vi "HandleObservation.vi"(8 "error in (no error)":errorcluster, 11 "S4ACS_GUI in":refnum<class "S4ACS_GUI.lvclass">) -> (0 "error out":errorcluster, 3 "S4ACS_GUI out":refnum<class "S4ACS_GUI.lvclass">)   [LabVIEW 2018, in "S4ACS_GUI.lvclass"]
uses:
  S4ACS_GUI.lvclass
  S4ACS_GUI.lvclass/S4ACS_GUI.ctl
  Server/Server.lvclass/Server.ctl
  Acquisition/Acquisition.lvclass
  C:/Users/observer/Desktop/Sparc4GUI/SPARC4_GUI/Server/Server.lvclass
  Server/Server.lvclass
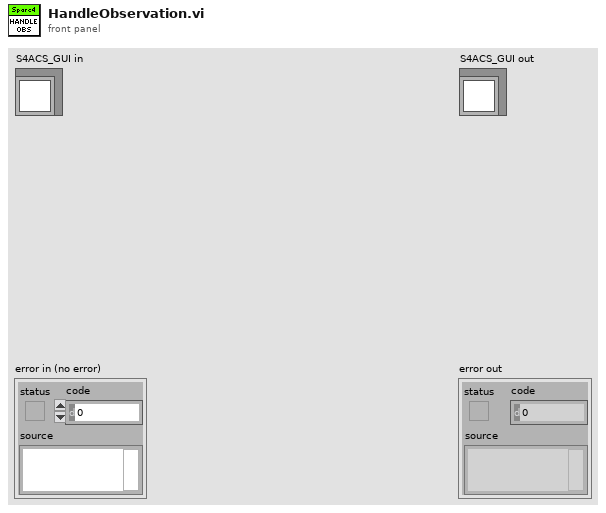
[diagram p1: front panel]
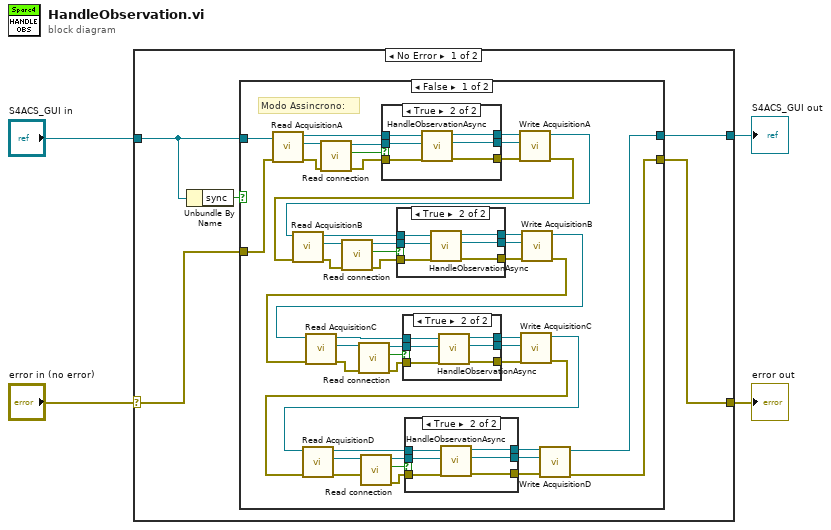
[diagram p0: block diagram]
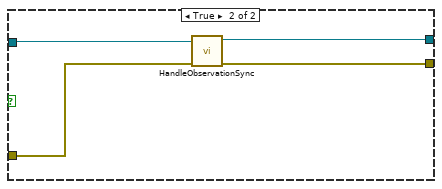
[diagram p6: hidden frame]
diagram:
  n1 = case shown="No Error" "error in (no error)" {
    selector: "error in (no error)" -> [w6 w97]
    tunnel: [w5 w97] -> w3
    tunnel: [w8 w96] -> w1
    tunnel: "S4ACS_GUI in" -> [w9 w96]
    frame No Error {
      n2 = Unbundle By Name(w9) -> ("sync"=w7:bool)
      n3 = case shown="False" w7 {
        tunnel: w9 -> [w55 w95]
        tunnel: [w47 w94] -> w8
        tunnel: w6 -> [w53 w93]
        tunnel: [w46 w92] -> w5
        frame False {
          # "Modo Assincrono:"
          n4 = call-dynamic "Read AcquisitionA.vi"("error in (no error)"=w53, "S4ACS_GUI in"=w55) -> ("error out"=w38:errorcluster, "Acquisition.lvclass"=w41:refnum<class "Acquisition.lvclass">, "S4ACS_GUI out"=w54:refnum<class "S4ACS_GUI.lvclass">)  [unwired: 7 in]
          n5 = call "Read connection.vi"("error in (no error)"=w38, "Server in"=w41) -> ("error out"=w37:errorcluster, "connection"=w39:bool, "Server out"=w40:refnum<class "Acquisition.lvclass">)  [unwired: 7 in]
          n6 = case shown="True" w39 {
            tunnel: w54 -> [w84 w91]
            tunnel: w40 -> [w85 w90]
            tunnel: w37 -> [w83 w89]
            tunnel: [w84 w88] -> w52
            tunnel: [w85 w87] -> w51
            tunnel: [w83 w86] -> w50
            frame False {
            }
            frame True {
              n7 = call-dynamic "HandleObservationAsync.vi"("error in (no error)"=w89, "Acquisition.lvclass In"=w90, "S4ACS_GUI in"=w91) -> ("error out"=w86:errorcluster, "Acquisition.lvclass Out"=w87:refnum<class "Acquisition.lvclass">, "S4ACS_GUI out"=w88:refnum<class "S4ACS_GUI.lvclass">)  [unwired: 6 in]
            }
          }
          n8 = call-dynamic "Write AcquisitionA.vi"("error in (no error)"=w50, "Acquisition.lvclass"=w51, "S4ACS_GUI in"=w52) -> ("error out"=w49:errorcluster, "S4ACS_GUI out"=w48:refnum<class "S4ACS_GUI.lvclass">)  [unwired: 7 in]
          n9 = call "Read AcquisitionB.vi"("error in (no error)"=w49, "S4ACS_GUI in"=w48) -> ("error out"=w32:errorcluster, "Acquisition.lvclass"=w35:refnum<class "Acquisition.lvclass">, "S4ACS_GUI out"=w36:refnum<class "S4ACS_GUI.lvclass">)  [unwired: 7 in]
          n10 = call "Read connection.vi"("error in (no error)"=w32, "Server in"=w35) -> ("error out"=w31:errorcluster, "connection"=w33:bool, "Server out"=w34:refnum<class "Acquisition.lvclass">)  [unwired: 7 in]
          n11 = case shown="True" w33 {
            tunnel: w36 -> [w75 w82]
            tunnel: w34 -> [w76 w81]
            tunnel: w31 -> [w74 w80]
            tunnel: [w75 w79] -> w28
            tunnel: [w76 w78] -> w29
            tunnel: [w74 w77] -> w30
            frame False {
            }
            frame True {
              n12 = call-dynamic "HandleObservationAsync.vi"("error in (no error)"=w80, "Acquisition.lvclass In"=w81, "S4ACS_GUI in"=w82) -> ("error out"=w77:errorcluster, "Acquisition.lvclass Out"=w78:refnum<class "Acquisition.lvclass">, "S4ACS_GUI out"=w79:refnum<class "S4ACS_GUI.lvclass">)  [unwired: 6 in]
            }
          }
          n13 = call "Write AcquisitionB.vi"("error in (no error)"=w30, "Acquisition.lvclass"=w29, "S4ACS_GUI in"=w28) -> ("error out"=w45:errorcluster, "S4ACS_GUI out"=w44:refnum<class "S4ACS_GUI.lvclass">)  [unwired: 7 in]
          n14 = call-dynamic "Read AcquisitionC.vi"("error in (no error)"=w45, "S4ACS_GUI in"=w44) -> ("error out"=w19:errorcluster, "Acquisition.lvclass"=w20:refnum<class "Acquisition.lvclass">, "S4ACS_GUI out"=w24:refnum<class "S4ACS_GUI.lvclass">)  [unwired: 7 in]
          n15 = call "Read connection.vi"("error in (no error)"=w19, "Server in"=w20) -> ("error out"=w25:errorcluster, "connection"=w26:bool, "Server out"=w27:refnum<class "Acquisition.lvclass">)  [unwired: 7 in]
          n16 = case shown="True" w26 {
            tunnel: w24 -> [w66 w73]
            tunnel: w27 -> [w67 w72]
            tunnel: w25 -> [w65 w71]
            tunnel: [w66 w70] -> w23
            tunnel: [w67 w69] -> w22
            tunnel: [w65 w68] -> w21
            frame False {
            }
            frame True {
              n17 = call-dynamic "HandleObservationAsync.vi"("error in (no error)"=w71, "Acquisition.lvclass In"=w72, "S4ACS_GUI in"=w73) -> ("error out"=w68:errorcluster, "Acquisition.lvclass Out"=w69:refnum<class "Acquisition.lvclass">, "S4ACS_GUI out"=w70:refnum<class "S4ACS_GUI.lvclass">)  [unwired: 6 in]
            }
          }
          n18 = call-dynamic "Write AcquisitionC.vi"("error in (no error)"=w21, "Acquisition.lvclass"=w22, "S4ACS_GUI in"=w23) -> ("error out"=w42:errorcluster, "S4ACS_GUI out"=w43:refnum<class "S4ACS_GUI.lvclass">)  [unwired: 7 in]
          n19 = call-dynamic "Read AcquisitionD.vi"("error in (no error)"=w42, "S4ACS_GUI in"=w43) -> ("error out"=w14:errorcluster, "Acquisition.lvclass"=w13:refnum<class "Acquisition.lvclass">, "S4ACS_GUI out"=w15:refnum<class "S4ACS_GUI.lvclass">)  [unwired: 7 in]
          n20 = call "Read connection.vi"("error in (no error)"=w14, "Server in"=w13) -> ("error out"=w16:errorcluster, "connection"=w17:bool, "Server out"=w18:refnum<class "Acquisition.lvclass">)  [unwired: 7 in]
          n21 = case shown="True" w17 {
            tunnel: w15 -> [w57 w64]
            tunnel: w18 -> [w58 w63]
            tunnel: w16 -> [w56 w62]
            tunnel: [w57 w61] -> w12
            tunnel: [w58 w60] -> w11
            tunnel: [w56 w59] -> w10
            frame False {
            }
            frame True {
              n22 = call-dynamic "HandleObservationAsync.vi"("error in (no error)"=w62, "Acquisition.lvclass In"=w63, "S4ACS_GUI in"=w64) -> ("error out"=w59:errorcluster, "Acquisition.lvclass Out"=w60:refnum<class "Acquisition.lvclass">, "S4ACS_GUI out"=w61:refnum<class "S4ACS_GUI.lvclass">)  [unwired: 6 in]
            }
          }
          n23 = call-dynamic "Write AcquisitionD.vi"("error in (no error)"=w10, "Acquisition.lvclass"=w11, "S4ACS_GUI in"=w12) -> ("error out"=w46:errorcluster, "S4ACS_GUI out"=w47:refnum<class "S4ACS_GUI.lvclass">)  [unwired: 7 in]
        }
        frame True {
          n24 = call-dynamic "HandleObservationSync.vi"("error in (no error)"=w93, "S4ACS_GUI in"=w95) -> ("error out"=w92:errorcluster, "S4ACS_GUI out"=w94:refnum<class "S4ACS_GUI.lvclass">)  [unwired: 8 in]
        }
      }
    }
    frame Error {
    }
  }
  "error out" <- w3
  "S4ACS_GUI out" <- w1
